vi "Get Cell.vi"(10 "Cell Address":string, 11 "Worksheet":refnum<k24>) -> ()   [LabVIEW 2024]
uses:
  C:/Users/tupp_js/.nuget/packages/documentformat.openxml/3.3.0/lib/net46/DocumentFormat.OpenXml.dll
  net46/DocumentFormat.OpenXml.dll
  C:/Users/tupp_js/Documents/LabVIEW Data/Open Xml LabVIEW/DocumentFormat.OpenXml.Framework.dll
  Documents/LabVIEW Data/Open Xml LabVIEW/DocumentFormat.OpenXml.Framework.dll
panel:
  out "Count":i32
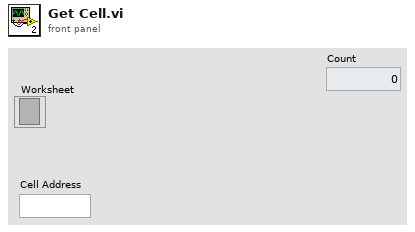
[diagram p1: front panel]
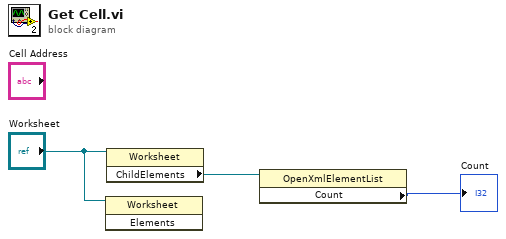
[diagram p0: block diagram]
diagram:
  n1 = invoke class="Worksheet" method="Elements"(reference="Worksheet") -> ()  [unwired: 2 in, 3 out]
  n2 = property class="Worksheet"(reference="Worksheet") -> ("ChildElements"=w2:refnum<k24>)  [unwired: 1 in, 2 out]
  n3 = property class="OpenXmlElementList"(reference=w2) -> ("Count"=→"Count":i32)  [unwired: 1 in, 2 out]
